vi "AlliGator Script Multi-ROI Single-Pixel Phasor Analysis.vi"(0 "Alligator Queue Elements in":T23[](array[typedef]), 1 "IRF File":path, 2 "Dataset File":path, 3 "ROI File":path, 5 "Error In":errorcluster, 6 "Phasor Graph refnum":refnum<vi>, 7 "Results Folder":path, 8 "Lifetime Graph Refnum":refnum<vi>, 10 "IRF Loading & Pre-processing Options":T4={"Data Information"={"Gates to Skip"={"Start"=0, "End"=0}, "# Gates"=1, "Gate Step"=1, "Gate Duration"=3e-10, "Gate Separation"=4e-11, "Pile-up Correction"=FALSE, "Pixel Well Capacity"=1, "Define Gates to"=enum."Skip", "Gates to Keep"={"First"=0, "Last"=0}, "Laser Period"=0.0, "SYNC Period"=0.0, "Channel Name"=0, "Channel Arithmetic"=enum."None", "Background File Subtraction"=FALSE, "Background Scaling Factor"=1.0, "Background File"=path "", "Background Pile-up Correction"=FALSE, "Background Pixel Well Capacity"=1, "Dataset Scaling Factor"=1.0}, "Source Image Settings"={"Low Count Pixels Rejection Options"={"Background Low Threshold Factor"=0.0, "Fixed Low Background Threshold"=20000.0, "Reject Low Count Pixels"=FALSE, "Low Percentile"=0.0}, "High Count Pixels Rejection Options"={"Background High Threshold Factor"=0.0, "Fixed High Background Threshold"=1.0, "Reject High Count Pixels"=FALSE, "High Percentile"=100.0}, "Peak Threshold"=500.0, "Intensity Threshold"=500.0, "Image Smoothing Options"={"Use Image Smoothing"=FALSE, "Kernel Type"=enum."Bilinear", "Bin"=1, "Algorithm"=enum."Rapid"}, "Image Binning Options"={"Use Image Binning"=FALSE, "X Bin"=1, "Y Bin"=1}}, "Decay Preprocessing Options & Parameters"={"Background Subtraction Parameters"={"Background Definition Range"={"Min Gate"=0.0, "Max Gate"=0.0}, "Baseline Subtraction Method"=enum."Mean", "Background Subtraction?"=FALSE, "Background File"=path "", "Background Constant"=0.0, "Background Scaling Factor"=1.0, "Background Pile-up Correction"=FALSE, "Background Pixel Well Capacity"=1}, "Decay Preprocessing Parameters"={"Background Subtraction"=FALSE, "Straighten Decay"=FALSE, "Reverse Gates"=FALSE, "1-Normalized Decay"=FALSE, "Smoothen Decay"=FALSE, "Smoothing Parameter"=0.0, "Shift Decay"=FALSE, "Decay Shift Parameters"={"Type"=enum."Default", "Shift"=0.0, "Threshold"=0.0, "Rotate"=FALSE}, "Extrapolate Decay"=FALSE, "Additional Points"=0, "Head Fraction"=0.0, "Pixel-Normalize Decay"=FALSE, "Use Periodicity"=FALSE, "Use Cursors"=FALSE, "Tail Fraction"=0.0, "Use Decay Pre-Processing"=TRUE, "Fold Decay"=FALSE, "# Folds"=1, "[0-1]-Normalized Decay"=FALSE}, "Preprocessing Steps Order"=[]}, "Clear Phasor Graph"=FALSE} {"Decay Preprocessing Options & Parameters"."Decay Preprocessing Parameters"."# Folds" min=1; "Decay Preprocessing Options & Parameters"."Background Subtraction Parameters"."Background Pixel Well Capacity" min=1 step=1; "Source Image Settings"."Image Binning Options"."Y Bin" min=1; "Source Image Settings"."Image Binning Options"."X Bin" min=1; "Source Image Settings"."Image Smoothing Options"."Bin" min=1; "Source Image Settings"."High Count Pixels Rejection Options"."High Percentile" min=0.0 max=100.0; "Source Image Settings"."Low Count Pixels Rejection Options"."Low Percentile" min=0.0 max=100.0; "Data Information"."Background Pixel Well Capacity" min=1 step=1; "Data Information"."Channel Name" items=["Bottom INT Gate", "Bottom G2 Gate"]; "Data Information"."SYNC Period" min=0.0 format="%#.3g"; "Data Information"."Laser Period" min=0.0 format="%#.3g"; "Data Information"."Pixel Well Capacity" min=1 step=1; "Data Information"."# Gates" min=1 step=1; "Data Information"."Gate Step" min=1 step=1; "Data Information"."Gate Duration" min=0.0 format="%#.3g"; "Data Information"."Gate Separation" min=0.0 format="%#.3g"}, 11 "Phasor Parameters Scatter Plot":T1[](array[typedef]), 12 "Dataset Loading & Pre-processing Options":T4={"Data Information"={"Gates to Skip"={"Start"=0, "End"=0}, "# Gates"=1, "Gate Step"=1, "Gate Duration"=3e-10, "Gate Separation"=4e-11, "Pile-up Correction"=FALSE, "Pixel Well Capacity"=1, "Define Gates to"=enum."Skip", "Gates to Keep"={"First"=0, "Last"=0}, "Laser Period"=0.0, "SYNC Period"=0.0, "Channel Name"=0, "Channel Arithmetic"=enum."None", "Background File Subtraction"=FALSE, "Background Scaling Factor"=1.0, "Background File"=path "", "Background Pile-up Correction"=FALSE, "Background Pixel Well Capacity"=1, "Dataset Scaling Factor"=1.0}, "Source Image Settings"={"Low Count Pixels Rejection Options"={"Background Low Threshold Factor"=0.0, "Fixed Low Background Threshold"=20000.0, "Reject Low Count Pixels"=FALSE, "Low Percentile"=0.0}, "High Count Pixels Rejection Options"={"Background High Threshold Factor"=0.0, "Fixed High Background Threshold"=1.0, "Reject High Count Pixels"=FALSE, "High Percentile"=100.0}, "Peak Threshold"=500.0, "Intensity Threshold"=500.0, "Image Smoothing Options"={"Use Image Smoothing"=FALSE, "Kernel Type"=enum."Bilinear", "Bin"=1, "Algorithm"=enum."Rapid"}, "Image Binning Options"={"Use Image Binning"=FALSE, "X Bin"=1, "Y Bin"=1}}, "Decay Preprocessing Options & Parameters"={"Background Subtraction Parameters"={"Background Definition Range"={"Min Gate"=0.0, "Max Gate"=0.0}, "Baseline Subtraction Method"=enum."Mean", "Background Subtraction?"=FALSE, "Background File"=path "", "Background Constant"=0.0, "Background Scaling Factor"=1.0, "Background Pile-up Correction"=FALSE, "Background Pixel Well Capacity"=1}, "Decay Preprocessing Parameters"={"Background Subtraction"=FALSE, "Straighten Decay"=FALSE, "Reverse Gates"=FALSE, "1-Normalized Decay"=FALSE, "Smoothen Decay"=FALSE, "Smoothing Parameter"=0.0, "Shift Decay"=FALSE, "Decay Shift Parameters"={"Type"=enum."Default", "Shift"=0.0, "Threshold"=0.0, "Rotate"=FALSE}, "Extrapolate Decay"=FALSE, "Additional Points"=0, "Head Fraction"=0.0, "Pixel-Normalize Decay"=FALSE, "Use Periodicity"=FALSE, "Use Cursors"=FALSE, "Tail Fraction"=0.0, "Use Decay Pre-Processing"=TRUE, "Fold Decay"=FALSE, "# Folds"=1, "[0-1]-Normalized Decay"=FALSE}, "Preprocessing Steps Order"=[]}, "Clear Phasor Graph"=FALSE} {"Decay Preprocessing Options & Parameters"."Decay Preprocessing Parameters"."# Folds" min=1; "Decay Preprocessing Options & Parameters"."Background Subtraction Parameters"."Background Pixel Well Capacity" min=1 step=1; "Source Image Settings"."Image Binning Options"."Y Bin" min=1; "Source Image Settings"."Image Binning Options"."X Bin" min=1; "Source Image Settings"."Image Smoothing Options"."Bin" min=1; "Source Image Settings"."High Count Pixels Rejection Options"."High Percentile" min=0.0 max=100.0; "Source Image Settings"."Low Count Pixels Rejection Options"."Low Percentile" min=0.0 max=100.0; "Data Information"."Background Pixel Well Capacity" min=1 step=1; "Data Information"."Channel Name" items=["Bottom INT Gate", "Bottom G2 Gate"]; "Data Information"."SYNC Period" min=0.0 format="%#.3g"; "Data Information"."Laser Period" min=0.0 format="%#.3g"; "Data Information"."Pixel Well Capacity" min=1 step=1; "Data Information"."# Gates" min=1 step=1; "Data Information"."Gate Step" min=1 step=1; "Data Information"."Gate Duration" min=0.0 format="%#.3g"; "Data Information"."Gate Separation" min=0.0 format="%#.3g"}) -> (14 "Alligator Queue Elements out":T23[](array[typedef]), 17 "Message":string, 19 "Error Out":errorcluster)   [LabVIEW 2021, in "AlliGator Scripts.lvlib"]
doc: "Scripts performing phasor analysis of all pixels in all ROIs, using individual IRFs if provided."
uses:
  AlliGator Scripts.lvlib
  Action Engine/AlliGator Q Event.ctl
  Action Engine/AlliGator Action Engine.lvlib
  Action Engine/AlliGator Q Element.ctl
  Action Engine/Alligator Elements Order in Action Stack.ctl
  Strings/Strings.lvlib
  Action Engine/AlliGator Add Action Array to Stack.vi
  Globals, Variables, Constants/AlliGator Globals, Variables & Constants.lvlib
  Globals, Variables, Constants/AlliGator Variables List.ctl
  Phasor/Phasor Calibration Type.ctl
  Phasor/Phasor.lvlib
  Files/Load-Save File Info.ctl
  Files/Files.lvlib
  <vilib>/Utility/miscctls.llb/LVPoint32TypeDef.ctl
  Graphs/XY Graph/XY Graph Refnum.ctl
  Graphs/XY Graph/XY Graph Add-Ons.lvlib
  Graphs/XY Graph/XY Graph Mouse Click Event Data.ctl
  Settings/AlliGator Settings.lvlib
  Action Engine/AlliGator Add Single Action to Stack.vi
  Graphs/XY Graph/XY Graph Save Plot Data.ctl
  Graphs/XY Graph/XY Graph Selected Plot Info.ctl
  Phasor Graph/AlliGator Phasor Graph.lvlib
  <vilib>/ErrorRing/Error Ring.xnode
  <vilib>/Utility/error.llb/Error Cluster From Error Code.vi
  ROIs/AlliGator ROIs.lvlib
  Graphs/Graphs.lvlib
  Settings/AlliGator Background Subtraction Parameters.ctl
  Settings/AlliGator Gates to Keep.ctl
  AlliGator Data Information.ctl
  Settings/AlliGator Low Count Pixels Rejection Options.ctl
  Settings/AlliGator High Count Pixels Rejection Options.ctl
  Arrays/Kernel Type.ctl
  Arrays/Arrays.lvlib
  Arrays/Smoothing Algorithm.ctl
  Settings/AlliGator Image Smoothing Options.ctl
  Source Image/AlliGator Image Binning Options.ctl
  Source Image/AlliGator Source Image.lvlib
  AlliGator Source Image Settings.ctl
  Decay Analysis/Decay Preprocessing/AlliGator Baseline Subtraction Method.ctl
  Decay Analysis/Decay Preprocessing/AlliGator Decay Preprocessing.lvlib
  Decay Analysis/Decay Preprocessing/AlliGator Background Subtraction Parameters.ctl
  Graphs/XY Graph/XY Graph Plot Shift Method.ctl
  Graphs/XY Graph/XY Graph Plot Shift Parameters.ctl
  Decay Analysis/Decay Preprocessing/AlliGator Decay Preprocessing Parameters.ctl
  Decay Analysis/Decay Preprocessing/AlliGator Decay Preprocessing Options.ctl
  AlliGator Data Load & Process Options.ctl
  Settings/AlliGator Gate Arithmetic.ctl
  Phasor Graph/AlliGator Phasor Graph Parameter List.ctl
  Phasor Graph/AlliGator Phasor Plot Scatter Plot Parameters.ctl
  Settings/AlliGator Define Gates to.ctl
panel:
  in  "Tab Control":T3(tab)
  # "see the AlliGator License on the block diagram (Ctrl+E or Window:Show Block Diagram)"
  # "vs"
  # "Gates Characteristics"
  # "Background File Subtraction"
  # "Gates Characteristics"
  # "Background File Subtraction"
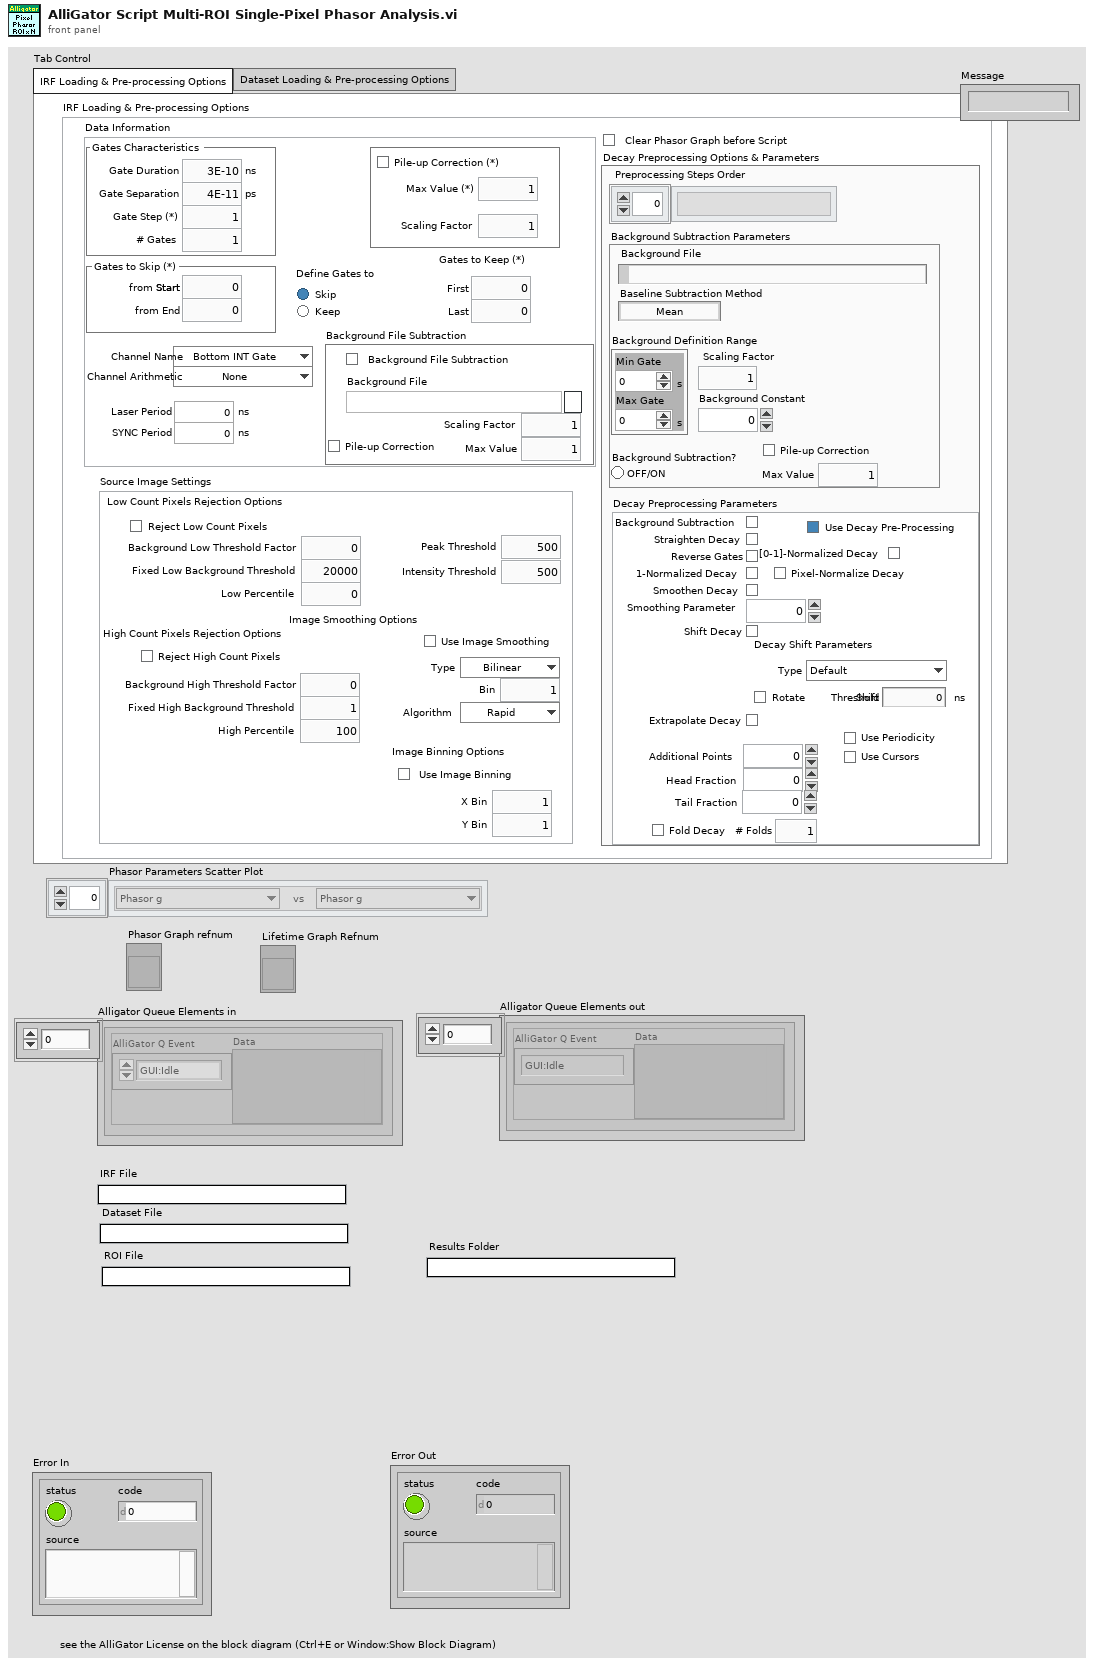
[diagram p1: front panel]
types:
  T1 = typedef "AlliGator Phasor Graph.lvlib/AlliGator Phasor Plot Scatter Plot Parameters.ctl" = cluster{"Parameter 2":T2, "Parameter 1":T2}
  T2 = typedef "AlliGator Phasor Graph.lvlib/AlliGator Phasor Graph Parameter List.ctl" = enum16{"Time Stamp", "Index", "Phasor Parameters", "Phasor g", "Phasor s", "Phasor phi", "Phasor m", "Modulus Lifetime", "Phase Lifetime", "ROI Parameters", "ROI Center x", "ROI Center y", "ROI # pixels ", "Decay Parameters", "Intensity", "Background/Gate", "Intensity - Background", "Fitted Lifetime", "Fitted Intensity", "Phasor Ratio Parameters", "Amplitude Phasor Ratio", "Intensity Phasor Ratio", "Amplitude-Averaged Lifetime", "Intensity-Averaged Lifetime", "-", "Phasor Parameters SDV", "Phasor g SDV", "Phasor s SDV", "Phasor phi SDV", "Phasor m SDV", "Phase Lifetime SDV", "Modulus Lifetime SDV", "Phasor Ratio Parameters SDV", "Amplitude Phasor Ratio SDV", "Intensity Phasor Ratio SDV", "Amplitude-Averaged Lifetime SDV", "Intensity-Averaged Lifetime SDV"}
  T3 = enum32{"IRF Loading & Pre-processing Options", "Dataset Loading & Pre-processing Options"}
  T4 = typedef "AlliGator Scripts.lvlib/AlliGator Data Load & Process Options.ctl" = cluster{"Data Information":T5, "Source Image Settings":T10, "Decay Preprocessing Options & Parameters":T17, "Clear Phasor Graph":bool}
  T5 = typedef "AlliGator Scripts.lvlib/AlliGator Data Information.ctl" = cluster{"Gates to Skip":T6, "# Gates":u32, "Gate Step":u32, "Gate Duration":dbl[unit], "Gate Separation":dbl[unit], "Pile-up Correction":bool, "Pixel Well Capacity":u32, "Define Gates to":T7, "Gates to Keep":T8, "Laser Period":dbl[unit], "SYNC Period":dbl[unit], "Channel Name":u16, "Channel Arithmetic":T9, "Background File Subtraction":bool, "Background Scaling Factor":dbl, "Background File":path, "Background Pile-up Correction":bool, "Background Pixel Well Capacity":u32, "Dataset Scaling Factor":dbl}
  T6 = typedef "AlliGator Settings.lvlib/AlliGator Background Subtraction Parameters.ctl" = cluster{"Start":u32, "End":u32}
  T7 = typedef "AlliGator Settings.lvlib/AlliGator Define Gates to.ctl" = enum32{"Skip", "Keep"}
  T8 = typedef "AlliGator Settings.lvlib/AlliGator Gates to Keep.ctl" = cluster{"First":u32, "Last":u32}
  T9 = typedef "AlliGator Settings.lvlib/AlliGator Gate Arithmetic.ctl" = enum16{"None", "INT-G2", "G2/INT*<INT>", "(1 - G2/INT)*<INT>"}
  T10 = typedef "AlliGator Scripts.lvlib/AlliGator Source Image Settings.ctl" = cluster{"Low Count Pixels Rejection Options":T11, "High Count Pixels Rejection Options":T12, "Peak Threshold":dbl, "Intensity Threshold":dbl, "Image Smoothing Options":T13, "Image Binning Options":T16}
  T11 = typedef "AlliGator Settings.lvlib/AlliGator Low Count Pixels Rejection Options.ctl" = cluster{"Background Low Threshold Factor":dbl, "Fixed Low Background Threshold":dbl, "Reject Low Count Pixels":bool, "Low Percentile":dbl}
  T12 = typedef "AlliGator Settings.lvlib/AlliGator High Count Pixels Rejection Options.ctl" = cluster{"Background High Threshold Factor":dbl, "Fixed High Background Threshold":dbl, "Reject High Count Pixels":bool, "High Percentile":dbl}
  T13 = typedef "AlliGator Settings.lvlib/AlliGator Image Smoothing Options.ctl" = cluster{"Use Image Smoothing":bool, "Kernel Type":T14, "Bin":i32, "Algorithm":T15}
  T14 = typedef "Arrays.lvlib/Kernel Type.ctl" = enum16{"Uniform", "Bilinear", "Gaussian"}
  T15 = typedef "Arrays.lvlib/Smoothing Algorithm.ctl" = enum16{"Rapid", "Thorough"}
  T16 = typedef "AlliGator Source Image.lvlib/AlliGator Image Binning Options.ctl" = cluster{"Use Image Binning":bool, "X Bin":i32, "Y Bin":i32}
  T17 = typedef "AlliGator Decay Preprocessing.lvlib/AlliGator Decay Preprocessing Options.ctl" = cluster{"Background Subtraction Parameters":T18, "Decay Preprocessing Parameters":T20, "Preprocessing Steps Order":string[]}
  T18 = typedef "AlliGator Decay Preprocessing.lvlib/AlliGator Background Subtraction Parameters.ctl" = cluster{"Background Definition Range":cluster{"Min Gate":dbl[unit], "Max Gate":dbl[unit]}, "Baseline Subtraction Method":T19, "Background Subtraction?":bool, "Background File":path, "Background Constant":dbl, "Background Scaling Factor":dbl, "Background Pile-up Correction":bool, "Background Pixel Well Capacity":u32}
  T19 = typedef "AlliGator Decay Preprocessing.lvlib/AlliGator Baseline Subtraction Method.ctl" = enum16{"Mean", "Min", "Square Gated Single-Exponential", "File", "Constant"}
  T20 = typedef "AlliGator Decay Preprocessing.lvlib/AlliGator Decay Preprocessing Parameters.ctl" = cluster{"Background Subtraction":bool, "Straighten Decay":bool, "Reverse Gates":bool, "1-Normalized Decay":bool, "Smoothen Decay":bool, "Smoothing Parameter":dbl, "Shift Decay":bool, "Decay Shift Parameters":T21, "Extrapolate Decay":bool, "Additional Points":u32, "Head Fraction":dbl, "Pixel-Normalize Decay":bool, "Use Periodicity":bool, "Use Cursors":bool, "Tail Fraction":dbl, "Use Decay Pre-Processing":bool, "Fold Decay":bool, "# Folds":u32, "[0-1]-Normalized Decay":bool}
  T21 = typedef "XY Graph Add-Ons.lvlib/XY Graph Plot Shift Parameters.ctl" = cluster{"Type":T22, "Shift":dbl[unit], "Threshold":dbl, "Rotate":bool}
  T22 = typedef "XY Graph Add-Ons.lvlib/XY Graph Plot Shift Method.ctl" = enum16{"Default", "CFD", "Threshold", "Cross-Correlation"}
  T23 = typedef "AlliGator Action Engine.lvlib/AlliGator Q Element.ctl" = cluster{"AlliGator Q Event":T24, "Data":variant}
  T24 = typedef "AlliGator Action Engine.lvlib/AlliGator Q Event.ctl" = enum16{"---- Files ----", "Files:Set Batch Export Files To Save", "Files:Set Dataset Loading & Pre-processing Options", "Files:Check #Frames in Dataset", "Files:Increment Frame Index", "Files:Open Mask Image", "Files:Open White Light Image", "Files:Open Single Dataset", "Files:New Folder of Folders Selected", "Files:Load File (all Types)_Scriptable", "Files:Move Flattened Series to Folders Series", "Files:Select Folder", "Files:Load FLI Dataset", "Files:Load Swiss SPAD 1 Dataset", "Files:Load Swiss SPAD 2 Dataset", "Files:Load .sdt FLI Dataset", "Files:Load .ptu FLI Dataset", "Files:Load .bin FLI Dataset", "Files:Load Single Gate Image Folder", "Files:Load I/m/phi Dataset (deprecated)", "Files:Load Single Image", "Files:Subtract Background File", "Files:Export FLI Dataset", "Files:Load HDF5 FLI Dataset", "Files:Set Destination File Path", "Files:Save Mask Image", "Files:Batch Conversion", "Files:New Folder Selected", "Files:Close FLI Dataset", "Files:Close FLI Dataset Series", "Files:Close White Light Image", "Files:Close Mask Image", "---- FLI Dataset ----", "FLI Dataset:Channel Arithmetic", "FLI Dataset:Export Average Lifetime Map as ASCII", "FLI Dataset:Export User-Defined Quantity Map as ASCII", "FLI Dataset:Python Function FLI Dataset Event", "FLI Dataset:ROI Analysis", "FLI Dataset:Tilted Logistic Square Gated IRF Characteristics Map", "FLI Dataset:Logistic Square Gated IRF Characteristics Map", "FLI Dataset:Square Gated IRF Characteristics Map", "FLI Dataset:Multi-ROI Single-Pixel Phasor Analysis", "FLI Dataset:Multi-ROI Single-Pixel NLSF Analysis", "FLI Dataset:All ROIs IRF Extraction", "FLI Dataset:All ROIs Decay Fit Non-Interactive (Fast + Individual IRF)", "FLI Dataset:All ROIs Phasor Analysis", "FLI Dataset:All ROIs Decay Fit", "FLI Dataset:Fluorescence Decay Statistics", "FLI Dataset:Update Decay Statistics Graph", "FLI Dataset:Get Decay from ROI", "FLI Dataset:All ROIs Average Lifetimes", "---- FLI Dataset Series ----", "FLI Dataset Series:Sum All Datasets in Series", "FLI Dataset Series:Add Dataset to Accumulated Dataset", "FLI Dataset Series:Display Accumulated Dataset", "FLI Dataset Series:Clear Dataset Series Sum", "FLI Dataset Series:Time-Series Analysis (NLSF)", "FLI Dataset Series:Time-Series Analysis (Phasor)", "---- Image ----", "Image:Update Image Profile Plots", "Image:Image Histogram Cursor Move", "Image:Image Histogram", "Image:Image Contrast", "Image:Set Image Histogram Cursor Move Flag", "Image:Clear Image Overlay", "Image:Use ROI as Search Area", "Image:Set ROI Diameter", "Image:Save Image Data as TIFF", "Image:Save Displayed Image with Overlay", "Image:Save Image Overlay Only", "Image:Save Image as Hot Pixel Mask", "Image:Change Source Image Color Palette", "Image:Copy Image to Clipboard", "Image:Source Image ROI Selection", "Image:Delete All ROIs", "Image:Delete All Unselected ROIs", "Image:Delete ROI", "Image:Merge All ROIs", "Image:Store ROI", "Image:Source Image ROI Storage", "Image:Export ROI Description to Notebook", "Image:Save ROI", "Image:Load ROI", "Image:Paste ROI Definition", "Image:Clear ROI", "Image:Identify ROIs in Mask Image", "Image:Create Complementary ROI", "Image:Create Contour ROI", "Image:Create ROI(s) from Pixels with Peak above Min_Scriptable", "Image:Create ROI(s) from Pixels with Intensity above Min_Scriptable", "Image:Compute ROI Statistics", "Image:Delete ROI(s) based on ROI Characteristics", "Image:Create ROI Grid", "Image:ROI to Individual Pixel ROIs", "Image:Python Function Source Image Event", "Image:Show Phasor Calibration Map ROI Centers", "Image:Convert ROI to Mask Image", "Image:Mouse Move", "Image:Mouse Up", "Image:Set Source Image Mouse Move Flag", "Image:Add Scale Bar Overlay", "Image:Delete Existing ROIs Option", "Image:Overlay ROI Median", "Image:Check Current ROI", "---- Decay ----", "Decay:Clear IRF/Reference Plot", "Decay:Clear Local IRFs", "Decay:Add Decay to Graph", "Decay:Smoothen Plot", "Decay:Smoothen Plot Tail", "Decay:Average Selected Plots", "Decay:Extract IRF", "Decay:Optimal IRF Extraction", "Decay:Threshold IRF", "Decay:Fit to Model IRF", "Decay:Fit IRF to Square Gate", "Decay:Fit IRF to Logistic Square Gate", "Decay:Fit IRF to Tilted Logistic Square Gate", "Decay:Create Bounding Cursors Set", "Decay:Export Bounding Cursors Definition to Notebook", "Decay:Denoise Plot", "Decay:Compute Cumulative Function", "Decay:Use as Reference Decay", "Decay:Show Reference Decay/IRF", "Decay:Extrapolate Decay", "Decay:Create Head & Tail Bounding Cursors", "Decay:Store Cursor-defined Head & Tail Fractions", "Decay:Rebin Plot", "Decay:1-Normalize Decay", "Decay:[0-1]-Normalize Plot", "Decay:Straighten Decay", "Decay:Shift Decay", "Decay:Fold Decay", "Decay:Fit Decay", "Decay:Global Fit of Selected Decays", "Decay:Post Global Fit Script", "Decay:Add Global Fit Parameters to Graph", "Decay:Add Decay Parameter(s) to Plot (Graph)", "Decay:Export Decay to Phasor Graph", "Decay:Plot Decay Shifts", "Decay:Compute Average Lifetime", "Decay:Plot Convolution", "Decay:Graph Tip Strip Update", "---- Decay Statistics ----", "Decay Statistics:Tip Strip Update", "---- Intensity Time Trace ----", "Intensity Time Trace:Use File Timestamp", "Intensity Time Trace:Load Intensity Corrections File", "Intensity Time Trace:Clear Intensity Corrections File", "Intensity Time Trace:Tip Strip Update", "---- Phasor Plot ----", "Phasor Plot:Build Phasor Plot", "Phasor Plot:Change Phasor Plot Color Palette", "Phasor Plot:Adjust Phasor Plot Display Range", "Phasor Plot:Highlight Image ROI in Phasor Plot", "Phasor Plot:Save Phasor Plot Image with Overlay", "Phasor Plot:Export Complex Phasor Map", "Phasor Plot:Export Phasor Ratio Map", "Phasor Plot:Export Average Lifetime Map", "Phasor Plot:Compute Phase Lifetime Histogram", "Phasor Plot:Compute Phasor Ratio Histogram", "Phasor Plot:Compute Phase Lifetime vs Intensity Scatter Plot", "Phasor Plot:Weber 2-Component Decomposition", "Phasor Plot:Update Phasor Color Map Vertices", "Phasor Plot:Clear Phasor Overlay", "Phasor Plot:Use Segment Extremities as References", "Phasor Plot:Use UC/Segment Intersections as References", "Phasor Plot:Use UC/Principal Axis Intersections as References", "Phasor Plot:Use UC/Linear Fit Intersections as References", "Phasor Plot:Update Phasor Plot Reference", "Phasor Plot:Show Local Phasor Info in Phasor Plot", "Phasor Plot:Update Phasor Plot State", "Phasor Plot:Phasor Plot ROI Storage", "Phasor Plot:Phasor Plot ROI Selection", "Phasor Plot:Python Function Phasor Plot Event", "Phasor Plot:Overlay Phasor ROI, Ratio or Map in Source Image", "Phasor Plot:Compute Decay of Selected Phasors", "Phasor Plot:Phasor at Image Pixel", "Phasor Plot:Mouse Move", "Phasor Plot:Mouse Up", "Phasor Plot:Display Range Mouse Move", "Phasor Plot:Set Mouse Move Flag", "---- Phasor Graph ----", "Phasor Graph:Calibrated Phasor Map Series", "Phasor Graph:Whole Image Phasor Scatter Plot (deprecated)", "Phasor Graph:Get Phasor Value", "Phasor Graph:Create New Phasor Plot Dialog", "Phasor Graph:Update Last Phasor Value", "Phasor Graph:Update Phasor (m, phi)", "Phasor Graph:Remove Single Phasor from Plot", "Phasor Graph:Add Single Phasor to Plot", "Phasor Graph:Remove Phasor Plot", "Phasor Graph:Remove Selected Phasor Plots", "Phasor Graph:Clear Phasor Data", "Phasor Graph:Clear Phasor Graph", "Phasor Graph:Cursor Move", "Phasor Graph:Draw Cursor Connecting Line", "Phasor Graph:Clear Cursor Connecting Line", "Phasor Graph:Find UC Intersection", "Phasor Graph:Use UC/Cursor-Defined Line Intersections", "Phasor Graph:Use Selected Plots Fitted Line/UC Intersections", "Phasor Graph:Use Selected Plots Principal Axis/UC Intersections", "Phasor Graph:Show Single Phasor", "Phasor Graph:Save Single Phasor Plot", "Phasor Graph:Save All Phasor Plots", "Phasor Graph:Load Phasor Plot(s)", "Phasor Graph:Phasor Multiplication", "Phasor Graph:Compute Average Phasor", "Phasor Graph:Compute Multiple Average Phasors (Selected Plots)", "Phasor Graph:Export Single Phasor Plot Phase Lifetimes", "Phasor Graph:Phase Lifetime Trajectory (deprecated)", "Phasor Graph:Phase Lifetime vs Intensity Scatter Plot (deprecated)", "Phasor Graph:Parameter 2 vs Parameter 1 Scatter Plot", "Phasor Graph:Use Cursor n Location", "Phasor Graph:Set Reference n to Current Phase Lifetime Value", "Phasor Graph:Set Reference n to Lifetime Value", "Phasor Graph:Set Cursor n Location", "Phasor Graph:Save Phasor Graph Image", "Phasor Graph:Update SEPL Plot", "Phasor Graph:Export Single Phasor Plot Data", "Phasor Graph:Export Selected Phasor Plots Data", "Phasor Graph:Python Function Phasor Graph Event", "Phasor Graph:Tip Strip Update", "---- Calibration ----", "Calibration:Set Calibration Type", "Calibration:Load/Save Phasor Calibration", "Calibration:Load/Save Phasor Calibration Series", "Calibration:Load/Save Phasor Calibration Map", "Calibration:Use as Calibration", "Calibration:Compute Optimal Calibration from Phasor References", "Calibration:Clear Phasor Calibration", "Calibration:Single Phasor Calibration Information", "Calibration:Use as Calibration Series", "Calibration:Use as Calibration Map", "Calibration:Clear Calibration Series", "Calibration:Phasor Calibration Series Information", "Calibration:Clear Calibration Map", "Calibration:Phasor Calibration Map Information", "Calibration:Apply Phasor Calibration", "Calibration:Update Single Plot Calibration", "Calibration:Update Multiple Plots Calibration", "Calibration:Clear Single Plot Calibration", "Calibration:Clear All Plots Calibrations", "Calibration:Clear Plot(s) Calibration(s)?", "Calibration:Phasor Calibration Maps (# Gates Series)", "---- Phasor Ratio ----", "Phasor Ratio:Clear Reference n", "Phasor Ratio:Toggle Selected Plot(s)  Lock to Reference 1", "Phasor Ratio:Use as Reference n", "Phasor Ratio:Send Reference n to Notebook", "Phasor Ratio:Toggle Selected Plot(s)  Lock to Reference 2", "Phasor Ratio:Compute Phasor Ratio at Mouse Location", "Phasor Ratio:Compute Phasor Plot's Average Phasor Ratio", "Phasor Ratio:Compute Time-Series Phasor Ratios", "Phasor Ratio:Fit Line to Phasor Ratio Plot", "Phasor Ratio:Save References", "Phasor Ratio:Load References", "Phasor Ratio:Update Phasor Reference 1", "Phasor Ratio:Update Phasor Reference 2", "Phasor Ratio:Move Cursor n to Reference n", "Phasor Ratio:Use as Phasor Reference 1 Lifetime", "Phasor Ratio:Use as Phasor Reference 2 Lifetime", "Phasor Ratio:Export Phasor Ratio Map as ASCII", "Phasor Ratio:Tip Strip Update", "---- Lifetime & Other Parameters Graph ----", "Lifetime:Tip Strip Update", "---- Decay Fit Parameter Map ----", "Decay Fit Parameter Map:Export ROI NLSF Data as ASCII", "Decay Fit Parameter Map:Set Decay Fit Parameter Map Selection", "Decay Fit Parameter Map:Build Decay Fit Parameter Map", "Decay Fit Parameter Map:Change Decay Fit Parameter Map Color Palette", "Decay Fit Parameter Map:Export Decay Fit Parameter Map Data as ASCII", "Decay Fit Parameter Map:Export All Decay Fit Parameter Maps Data as ASCII", "Decay Fit Parameter Map:Selected Parameter Scatterplot", "Decay Fit Parameter Map:Parameter 2 vs Parameter 1 Scatterplot", "Decay Fit Parameter Map:Save Decay Fit Parameter Map Image", "Decay Fit Parameter Map:Save-Load IRFs & Fit Data", "Decay Fit Parameter Map:Update Local Decay Plots", "Decay Fit Parameter Map:Python Function Decay Fit Parameters Map Event", "Decay Fit Parameter Map:Overlay Decay Fit Parameter Map in Source Image", "Decay Fit Parameter Map:Selected Parameter vs Intensity Scatterplot", "Decay Fit Parameter Map:Mouse Up", "Decay Fit Parameter Map:Display Range Mouse Move", "---- Parameter Map ----", "Parameter Map:Export ROI Parameters Data as ASCII", "Parameter Map:Delete Parameter Map Set", "Parameter Map:Update Parameter List", "Parameter Map:Build Parameter Map", "Parameter Map:Change Parameter Map Color Palette", "Parameter Map:Export Parameter Map Data as ASCII", "Parameter Map:Export All Parameter Maps Data as ASCII", "Parameter Map:Selected Parameter Scatterplot", "Parameter Map:Parameter 2 vs Parameter 1 Scatterplot", "Parameter Map:Selected Parameter vs Intensity Scatterplot", "Parameter Map:Save Parameter Map Image", "Parameter Map:Save-Load IRFs & Parameter Maps (TODO)", "Parameter Map:Set Parameter Map Selection", "Parameter Map:Python Function Parameter Map Event", "Parameter Map:Overlay Parameter Map in Source Image", "Parameter Map:Update Local Decay Plots", "Parameter Map:Mouse Up", "Parameter Map:Display Range Mouse Move", "---- Generic Graph ----", "Generic Graph:Generic XY Graph Event", "Generic Graph:Python Function XY Graph Event", "Generic Graph:New Plot", "Generic Graph:Save Plot", "Generic Graph:XY Plot Histogram", "Generic Graph:Set XY Graph Plot Name", "Generic Graph:Set Last Cursor Style", "Generic Graph:Tip Strip Update", "---- GUI ----", "GUI:Start Script", "GUI:Type of Displayed Image Changed", "GUI:Gate Image Slide Changed", "GUI:Show Busy Icon", "GUI:Show Busy Icon & Abort Button", "GUI:Hide Busy Icon", "GUI:Hide Busy Icon & Abort Button", "GUI:Abort", "GUI:End Script", "GUI:Start Timing", "GUI:End Timing", "GUI:Set State Indicator", "GUI:Send Parameters JSON Strings to Clipboard", "GUI:Set Gate Step", "GUI:Idle", "GUI:Initialization", "GUI:Quit", "GUI:Increment Dataset Index", "GUI:Set Dataset Index to -1", "GUI:Time Series Slider Moved", "GUI:Time Series Slider Changed", "GUI:Toggle Playback or Loop", "GUI:Playback Script", "GUI:Set Phasor Frequency", "GUI:Open Window", "GUI:Start Test Script", "GUI:End Test Script", "DEBUG"}
  T25 = typedef "AlliGator Globals, Variables & Constants.lvlib/AlliGator Variables List.ctl" = enum16{"---- GUI ----", "GUI:Initialization Status", "GUI:State Indicators Refnum", "GUI:Original AlliGator Menu Items", "GUI:Current Action Loop State", "GUI:Script in progress", "GUI:Playback", "GUI:Loop Playback", "GUI:Search ROI Used", "GUI:Search ROI", "Decay Graph Max Legend Size", "Intensity Graph Max Legend Size", "Decay Statistics Graph Max Legend Size", "Phasor Graph Max Legend Size", "Phasor Ratio Graph Max Legend Size", "Lifetime Graph Max Legend Size", "---- Files ----", "Files:Export Dataset Frames as Individual Files", "Files:Show Batch Export Help Balloons", "Files:Frames in Dataset", "Files:ptu File Frame Start Indices", "Files:Current Frame in Dataset", "Files:Current Frame Timestamp", "Files:Dataset Loaded", "Files:Dataset Metadata", "Files:Dataset Channel", "Files:Dataset Data Description", "Files:Background Dataset Metadata", "Files:Background Dataset Channel", "Files:Background Dataset Data Description", "Files:Background File Subtraction", "Files:Background File Path", "Files:Background File Pile-up Correction", "Files:Background File Pixel Well Capacity", "Files:Background File Scaling Factor", "Files:Current Dataset Load Settings", "Files:Dataset Path", "Files:ICCD-specific Information", "Files:Macrotime Gate Separation", "------ Python Plugins ------", "Python Plugins:Information", "Python Plugins:Python Session", "Python Plugins:Valid Python Session?", "---- Source Image ----", "Source Image:ROIs", "Source Image:Current ROI", "Source Image:ROI Event Refnum", "X_Source Image Display Range", "X_Source Image Palette Information", "X_Type of Displayed Image", "X_Time Gate Slider", "Source Image:Palette List", "Source Image:Scale", "Source Image:ROI Overlay Color", "Source Image:Overlay to Erase", "Source Image:Is Displayed Image Accumulated", "Source Image:White Light Image Modified", "Source Image:Mask Image Modified", "---- Image Profile Window ----", "Image Profile:Window Event Refnum", "Image Profile:IntensityType", "Image Profile:Intensity Average Type", "Image Profile:Intensity-weighted SDV", "Image Profile:Box Profile Type", "Image Profile:Window Open", "Image Profile:Plotted Fit Parameter", "------ Phasor Graph -------", "Phasor Graph:Show Line", "---- Phasor Plot ---", "Phasor Plot:Parameters Changed", "Phasor Plot:FLI Dataset Modified since last Calculation", "Phasor Harmonics Data", "Selected Phasor Harmonics", "Phasor Harmonic Manager Event Refnum", "Phasor Plot:ROIs", "Phasor Plot:Current ROI", "Phasor Plot:ROI Event Refnum", "Phasor Plot:Image Reference Points", "Phasor Plot:Computed", "Phasor Plot:Palette Information", "Phasor Plot:Palette List", "Phasor Plot:Phasor Ratio Palette Information", "Phasor Plot:Phasor Ratio Palette List", "Phasor Plot:Image Scale", "Phasor Plot:Image Overlay to Erase", "Phasor Plot:Image Elements to Update", "Phasor Plot:Current Calculation Parameters", "Phasor Plot:Current Calibration Options", "Phasor Plot:Reset Cumulated Phasor Plot", "Phasor Plot:Reference 1", "Phasor Plot:Lifetime Reference 1", "Phasor Plot:Reference 1 Frequency", "Phasor Plot:Reference 2", "Phasor Plot:Lifetime Reference 2", "Phasor Plot:Reference 2 Frequency", "---- Decay Analysis ----", "Number of Selected Decays to Fit", "LS Fit Results", "LAR Fit Results", "BS Fit Results", "Last Decay Max - Min", "Best Fit Parameters", "Best Fit Parameter Names", "Actual Size X", "Actual Size Y", "Binning X", "Binning Y", "Actual # Gates", "Dataset Number", "Gates to...", "Gates Skipped", "Gates to keep", "Gate Step", "Gate Separation", "Reversed Gates", "Pile-up Correction", "Pixel Well Capacity", "Background Subtracted", "Background Subtraction Method", "Background Definition Range", "Background File (deprecated)", "Number of Dataset Accumulated", "Array of Accumulated Dataset Paths", "Do Averaged Datasets", "Destination File Path", "Process Plot Target", "Use 1/D as Phasor Frequency", "---- Decay Fit Parameter Map -----", "Decay Fit Parameter Map:Palette Information", "Decay Fit Parameter Map:Palette List", "---- Parameter Map ----", "Parameter Map:Palette Information", "Parameter Map:Palette List", "------- Local Decay Window ---------", "Local Decay Graph Window:Event Refnum", "Local Decay Graph Window:Use normalized IRF for convolution", "----- Miscellaneous ----", "Misc:Skippable Dialog Windows Status"}
  T26 = enum16{"Start Script", "Load & Analyze IRF Dataset", "Load & Analyse FLI Dataset: Phasor", "End Script"}
  T27 = typedef "AlliGator Action Engine.lvlib/Alligator Elements Order in Action Stack.ctl" = enum16{"Enqueue 2 AFTER 1", "Enqueue 2 BEFORE 1"}
  T28 = typedef "Phasor.lvlib/Phasor Calibration Type.ctl" = enum16{"None", "Single Phasor", "Phasor Series", "Phasor Map"}
  T29 = typedef "XY Graph Add-Ons.lvlib/XY Graph Mouse Click Event Data.ctl" = cluster{"Multiplot XY Graph":T30, "Mouse Coordinates":T31}
  T30 = typedef "XY Graph Add-Ons.lvlib/XY Graph Refnum.ctl" = refnum<vi>
  T31 = typedef "LVPoint32TypeDef.ctl" = cluster{"Horizontal":i32, "Vertical":i32}
  T32 = typedef "XY Graph Add-Ons.lvlib/XY Graph Selected Plot Info.ctl" = cluster{"Multiplot XY Graph":T30, "Mouse Coordinates":T31, "Plot Index":i32}
  T33 = typedef "XY Graph Add-Ons.lvlib/XY Graph Save Plot Data.ctl" = cluster{"XY Graph Refnum":refnum<vi>, "Mouse Coords":T31, "File Path":path}
  T34 = typedef "Files.lvlib/Load-Save File Info.ctl" = cluster{"Load/Save":bool, "File Path":path}
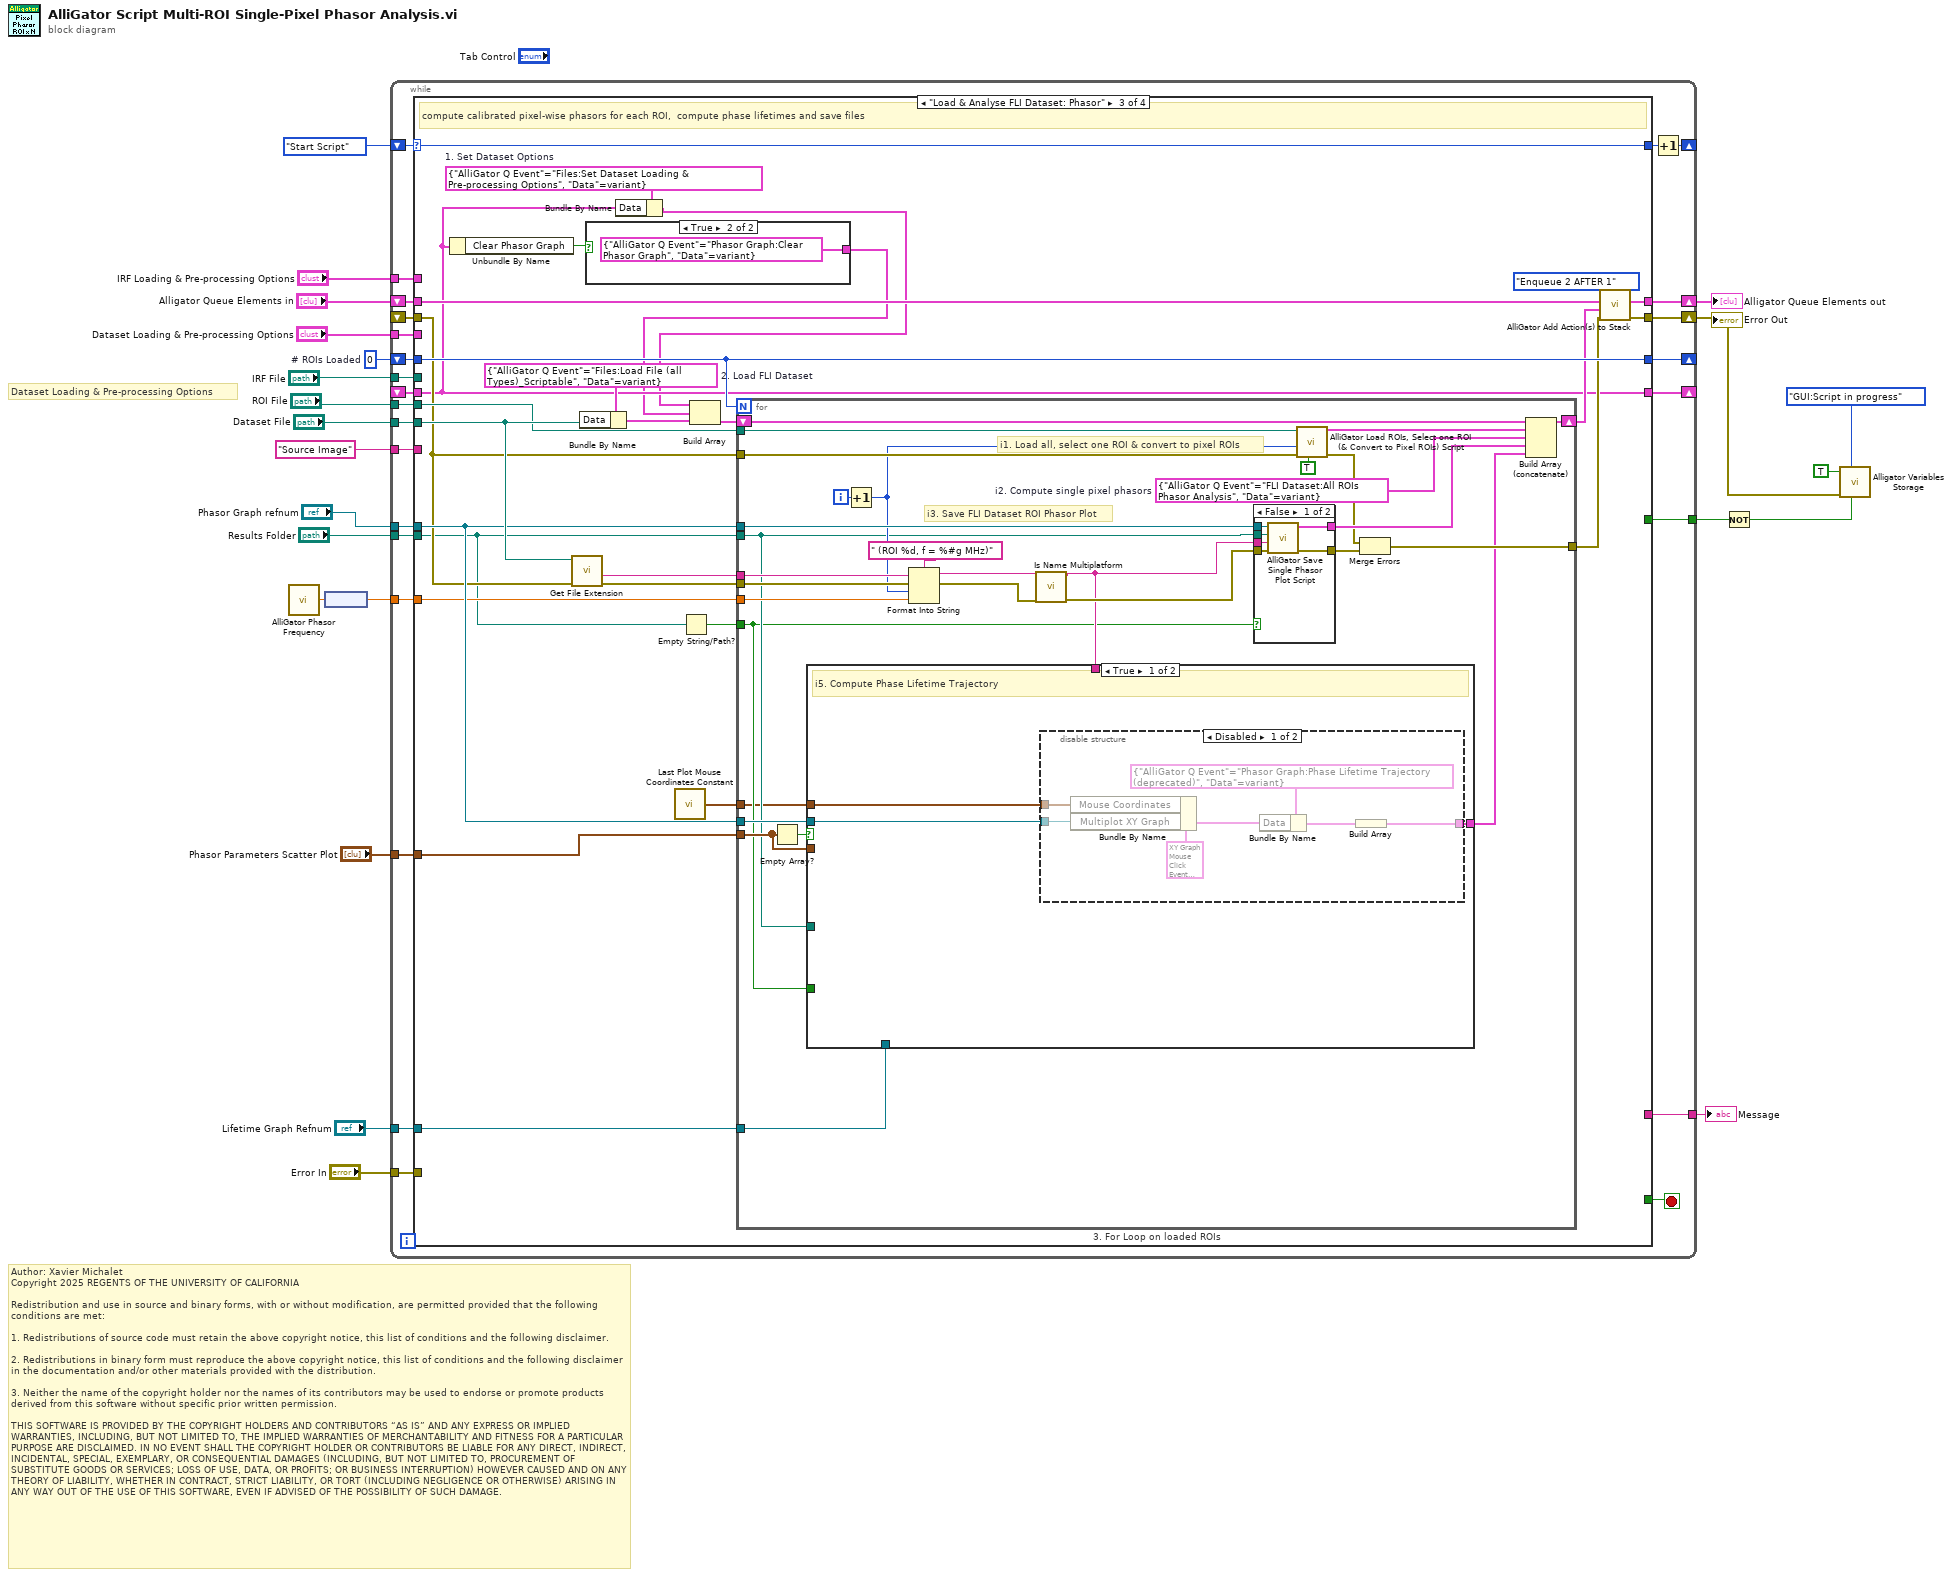
[diagram p0: block diagram]
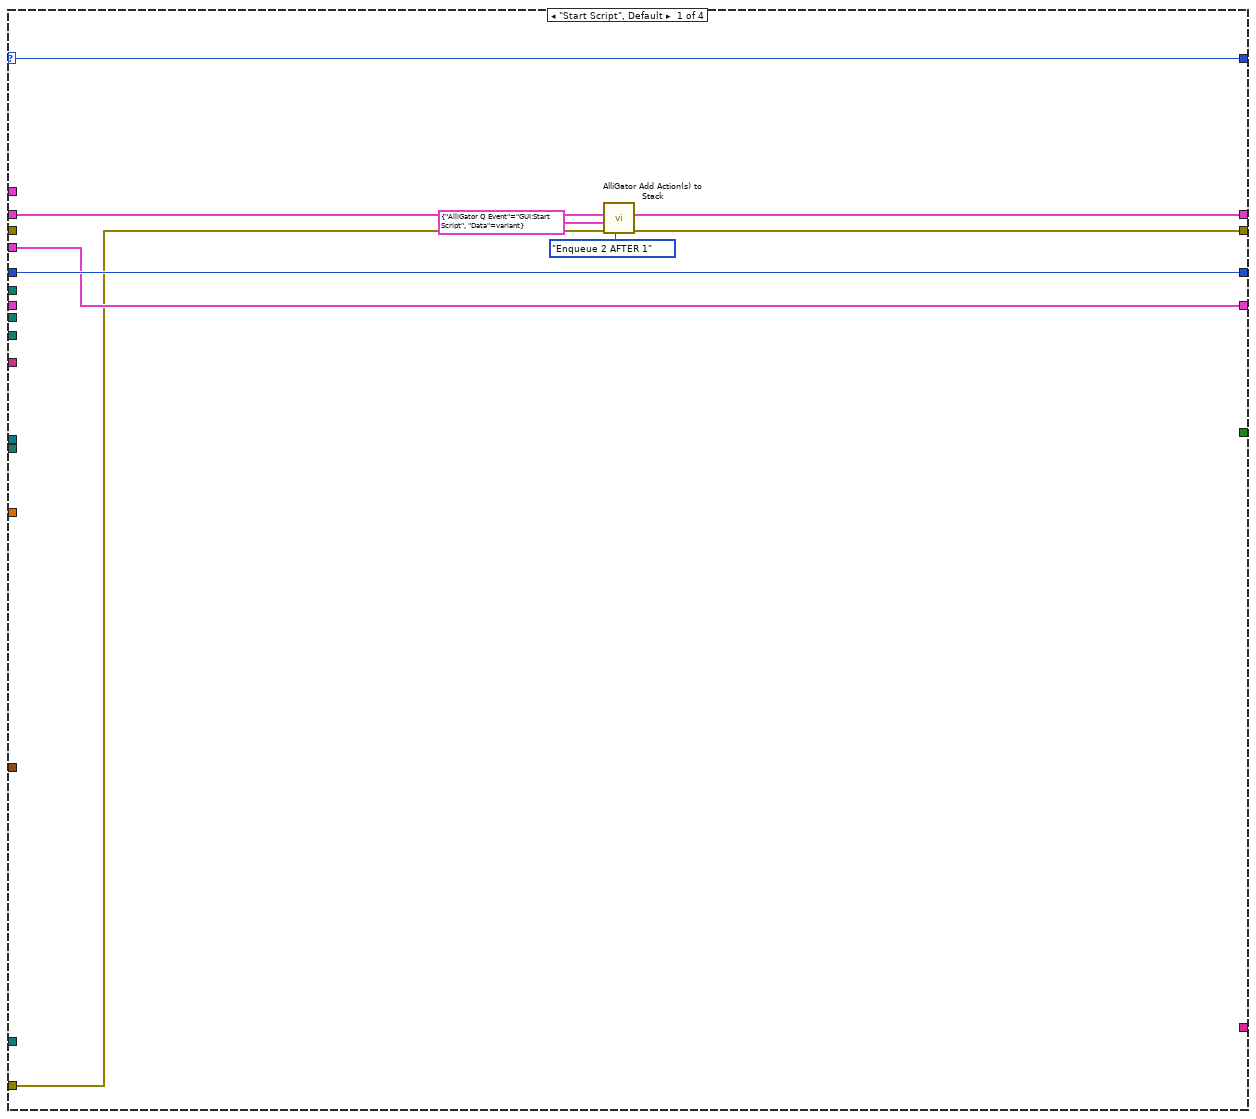
[diagram p2: hidden frame]
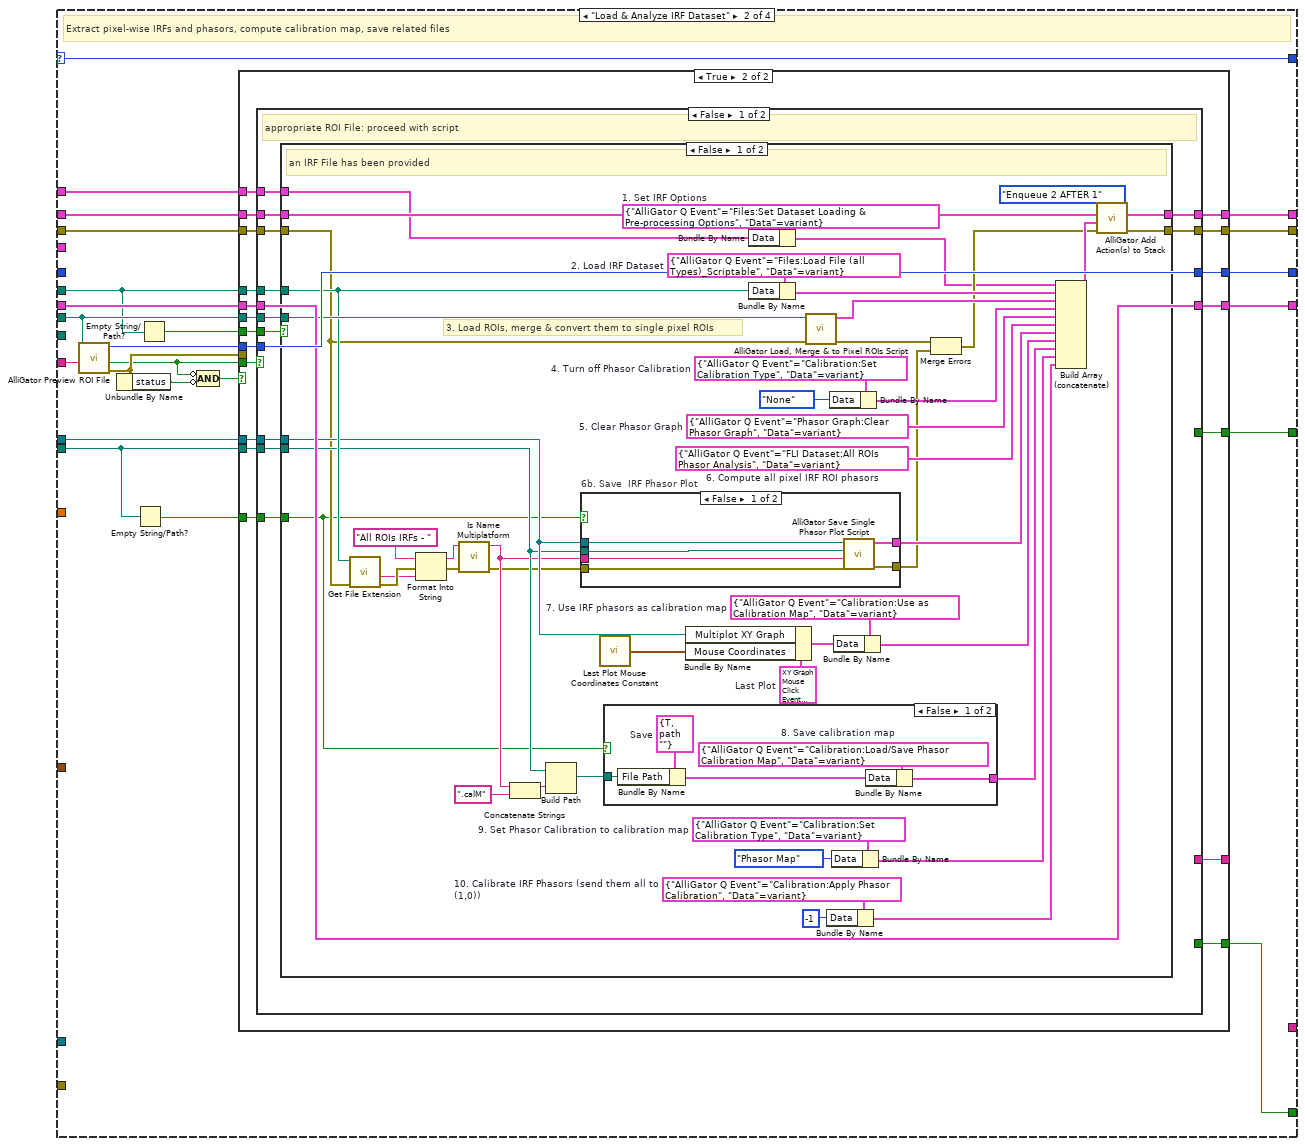
[diagram p3: hidden frame]
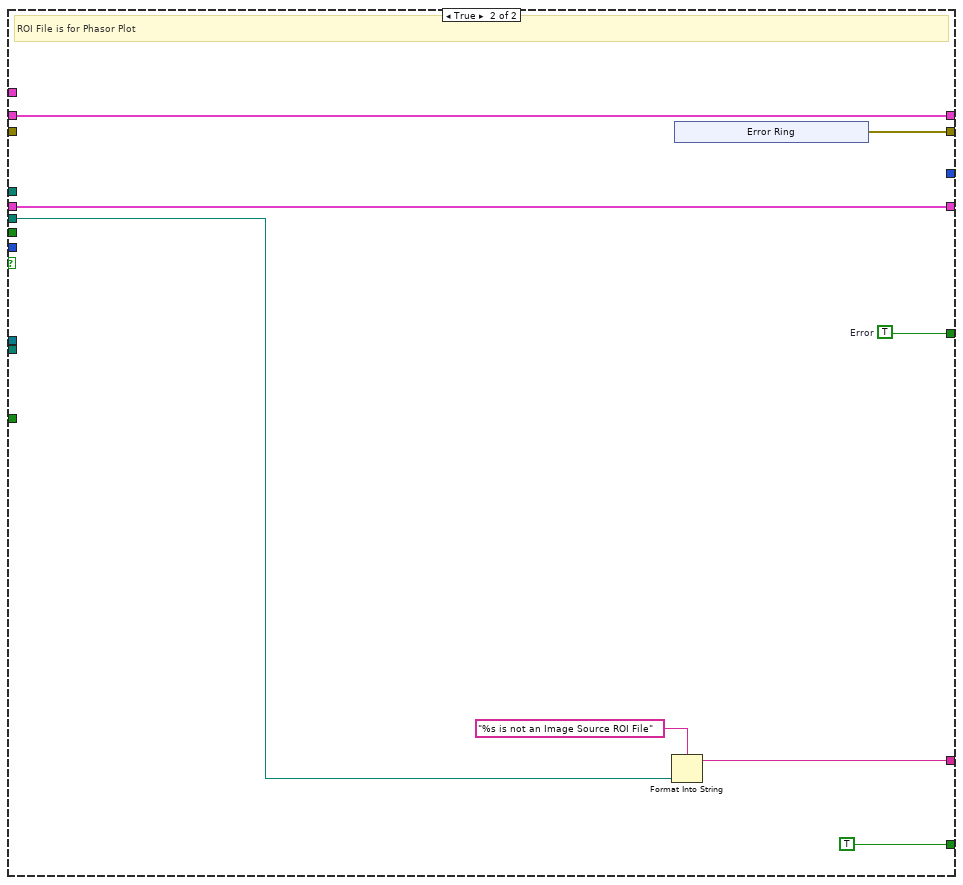
[diagram p8: hidden frame]
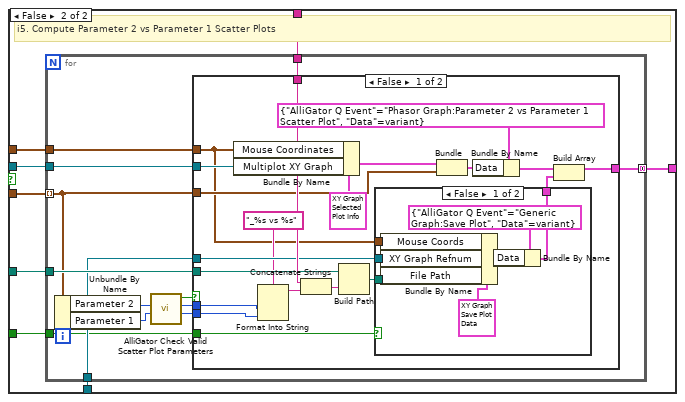
[diagram p11: hidden frame]
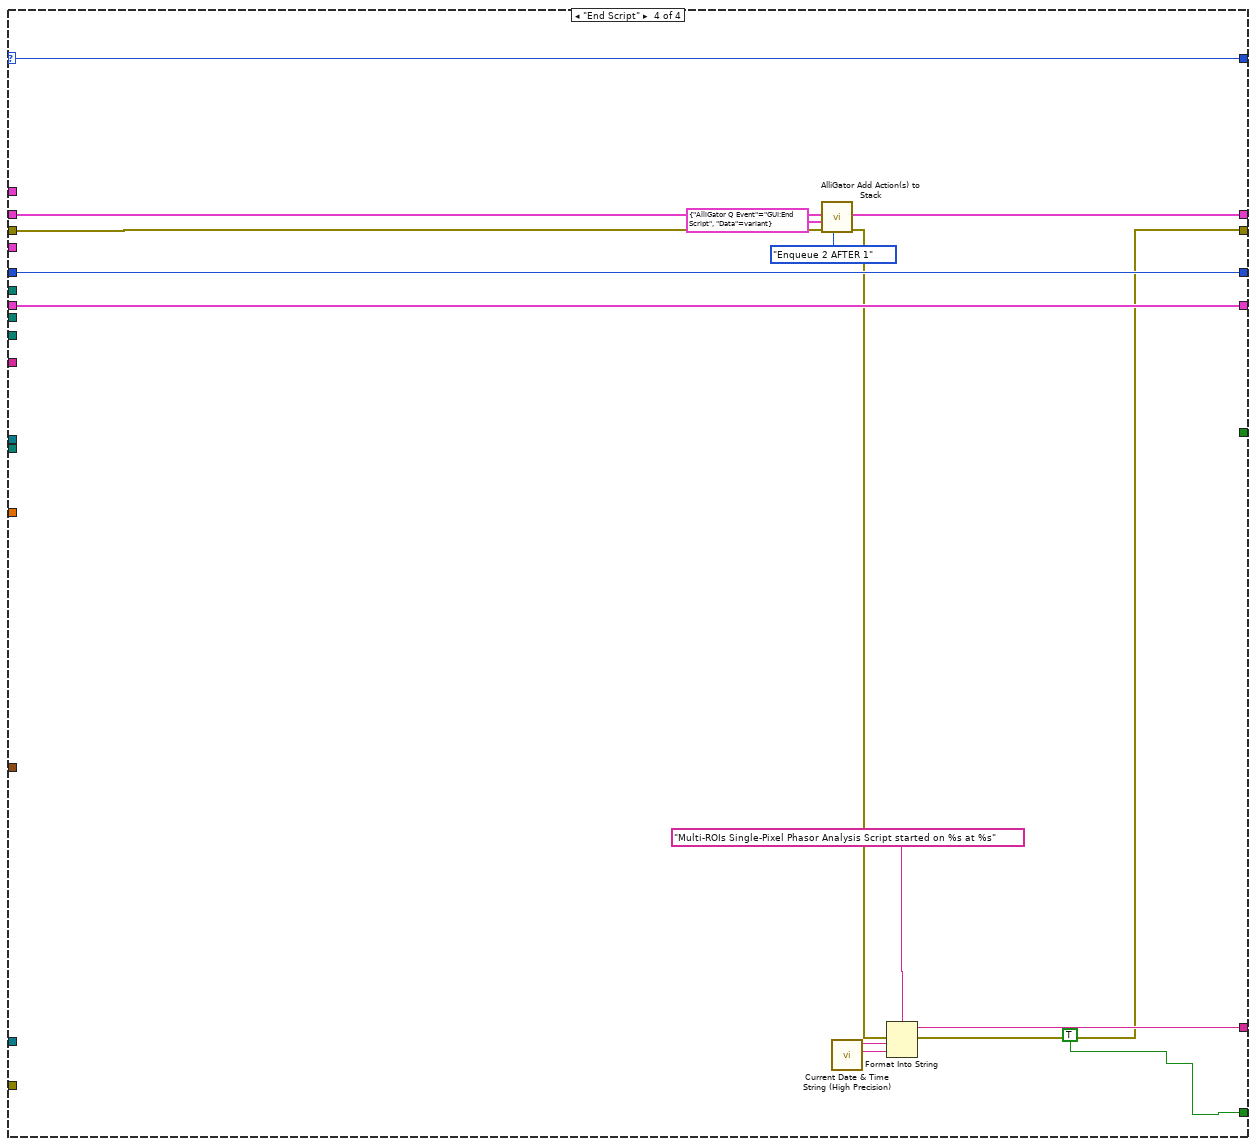
[diagram p15: hidden frame]
diagram:
  w10 = 0  # # ROIs Loaded
  # "Author: Xavier Michalet\nCopyright 2025 REGENTS OF THE UNIVERSITY OF CALIFORNIA\n\nRedistribution and use in source and binary forms, with or without modification, are permitted provided that the following conditions are met:\n\n1. Redistributions of source code must retain the above copyright notice, this list of conditions and the following disclaimer.\n\n2. Redistributions in binary form must reproduce the above copyright notice, this list of conditions and the following disclaimer in the documentation and/or other materials provided with the distribution.\n\n3. Neither the name of the copyright holder nor the names of its contributors may be used to endorse or promote products derived from this software without specific prior written permission.\n\nTHIS SOFTWARE IS PROVIDED BY THE COPYRIGHT HOLDERS AND CONTRIBUTORS “AS IS” AND ANY EXPRESS OR IMPLIED WARRANTIES, INCLUDING, BUT NOT LIMITED TO, THE IMPLIED WARRANTIES OF MERCHANTABILITY AND FITNESS FOR A PARTICULAR PURPOSE ARE DISCLAIMED. IN NO EVENT SHALL THE COPYRIGHT HOLDER OR CONTRIBUTORS BE LIABLE FOR ANY DIRECT, INDIRECT, INCIDENTAL, SPECIAL, EXEMPLARY, OR CONSEQUENTIAL DAMAGES (INCLUDING, BUT NOT LIMITED TO, PROCUREMENT OF SUBSTITUTE GOODS OR SERVICES; LOSS OF USE, DATA, OR PROFITS; OR BUSINESS INTERRUPTION) HOWEVER CAUSED AND ON ANY THEORY OF LIABILITY, WHETHER IN CONTRACT, STRICT LIABILITY, OR TORT (INCLUDING NEGLIGENCE OR OTHERWISE) ARISING IN ANY WAY OUT OF THE USE OF THIS SOFTWARE, EVEN IF ADVISED OF THE POSSIBILITY OF SUCH DAMAGE."
  # "Dataset Loading & Pre-processing Options"
  n1 = call "AlliGator Phasor Frequency.vi"() -> ("Phasor Frequency"=w7:dbl[unit])
  n2 = node(w7) -> (w8:dbl)
  n3 = while {
    shift-right: [w46] -> w13
    shift-left: _ -> [w49]
    shift-right: [w44] -> _
    shift-left: T26."Start Script" -> [w47]
    shift-right: [w42] -> w21
    shift-left: "Alligator Queue Elements in" -> [w48]
    tunnel: "IRF File" -> [w41]
    tunnel: "Phasor Graph refnum" -> [w40]
    tunnel: "ROI File" -> [w39]
    tunnel: "Dataset File" -> [w38]
    tunnel: "Source Image" ("Destination Image") -> [w37]
    shift-right: [w36] -> _
    shift-left: w10 -> [w34]
    tunnel: [w35] -> w12
    tunnel: "Results Folder" -> [w33]
    tunnel: w8 -> [w32]
    tunnel: "Lifetime Graph Refnum" -> [w31]
    tunnel: "Error In" -> [w30]
    shift-right: [w28] -> _
    shift-left: _ -> [w29]
    tunnel: "IRF Loading & Pre-processing Options" -> [w27]
    tunnel: "Dataset Loading & Pre-processing Options" -> [w26]
    tunnel: "Phasor Parameters Scatter Plot" -> [w25]
    tunnel: [w24] -> w1
    stop <- w43 stop-if-true
    n4 = case shown="\"Load & Analyse FLI Dataset: Phasor\"" w47 {
      selector: w47 -> [w58 w80 w216 w327]
      tunnel: w49 -> [_ w75 w207 w324]
      tunnel: w48 -> [w55 w81 w217 w325]
      tunnel: [w52 w78 w214 w314] -> w46
      tunnel: [w58 w80 w216 w327] -> w45
      tunnel: [_ w71 _ TRUE] -> w43
      tunnel: [w53 w79 w215 w323] -> w42
      tunnel: w41 -> [_ w65 _ _]
      tunnel: w40 -> [_ w77 w212 _]
      tunnel: w39 -> [_ w76 w211 _]
      tunnel: w38 -> [_ _ w213 _]
      tunnel: w37 -> [_ w74 _ _]
      tunnel: [w57 w72 w210 w318] -> w36
      tunnel: [_ w70 _ _] -> w35
      tunnel: w34 -> [w57 _ w210 w318]
      tunnel: w33 -> [_ w62 w196 _]
      tunnel: w32 -> [_ _ w209 _]
      tunnel: w31 -> [_ _ w208 _]
      tunnel: w30 -> [w54 _ _ _]
      tunnel: w29 -> [_ w69 w194 w317]
      tunnel: [w56 w68 w194 w317] -> w28
      tunnel: w27 -> [_ w67 _ _]
      tunnel: w26 -> [w56 _ _ _]
      tunnel: w25 -> [_ _ w197 _]
      tunnel: [_ _ _ w316] -> w24
      frame "Start Script", Default {
        n5 = call-poly "AlliGator Add Action(s) to Stack.vi"("Elements Order in Action Stack (Default: 2 BEFORE 1)"=Alligator_Elements_Order_in_Action_Stack."Enqueue 2 AFTER 1", "Error In"=w54, "Alligator Atomic Action"=T23 {"AlliGator Q Event"=enum."GUI:Start Script", "Data"=variant}, "Alligator Queue Element 1"=w55) -> ("Error Out"=w52:errorcluster, "Alligator Queue Element 1 (+ 2)"=w53:T23[])  [unwired: 6 in]
      }
      frame "Load & Analyze IRF Dataset" {
        # "Extract pixel-wise IRFs and phasors, compute calibration map, save related files"
        n6 = call "AlliGator Preview ROI File.vi"("Destination Image"=w74, "File Path"=w76) -> ("Error Out"=w63:errorcluster, "Phasor Plot Image"=w60:bool, "# ROIs Loaded"=w73:i32)  [unwired: 7 in]
        n7 = Unbundle By Name(w63) -> ("status"=w64:bool)
        n8 = Empty String/Path?(string/path=w62) -> (empty?=w61:bool)
        n9 = Empty String/Path?(string/path=w65) -> (empty?=w59:bool)
        n10 = Compound Arithmetic op=AND(invert w60, invert w64) -> (w66:bool)
        n11 = case shown="True" w66 {
          tunnel: w81 -> [w84 w103]
          tunnel: [w84 w102] -> w79
          tunnel: [w82 w101] -> w78
          tunnel: w77 -> [_ w100]
          tunnel: w76 -> [_ w99]
          tunnel: w75 -> [_ w98]
          tunnel: w65 -> [_ w97]
          tunnel: w73 -> [_ w95]
          tunnel: w60 -> [_ w96]
          tunnel: [_ w94] -> w72
          tunnel: [_ w93] -> _
          tunnel: [_ w92] -> w71
          tunnel: [_ w91] -> w70
          tunnel: w62 -> [_ w90]
          tunnel: w69 -> [w83 w89]
          tunnel: [w83 w88] -> w68
          tunnel: w67 -> [_ w87]
          tunnel: w63 -> [w82 _]
          tunnel: w61 -> [_ w86]
          tunnel: w59 -> [_ w85]
          frame False {
            # "Either error in or Phasor Plot Image ROIs"
          }
          frame True {
            n12 = case shown="False" w96 {
              tunnel: w103 -> [w116 w185]
              tunnel: [w115 w185] -> w102
              tunnel: [w114 w179] -> w101
              tunnel: w100 -> [w110 _]
              tunnel: w99 -> [w113 w183]
              tunnel: w98 -> [w108 _]
              tunnel: w97 -> [w112 _]
              tunnel: w95 -> [w111 _]
              tunnel: [w111 _] -> w94
              tunnel: [_ w184] -> w93
              tunnel: [_ TRUE] -> w92
              tunnel: [_ w180] -> w91
              tunnel: w90 -> [w109 _]
              tunnel: w89 -> [w106 w178]
              tunnel: [w106 w178] -> w88
              tunnel: w87 -> [w107 _]
              tunnel: w86 -> [w105 _]
              tunnel: w85 -> [w104 _]
              frame False {
                # "appropriate ROI File: proceed with script"
                n13 = case shown="False" w104 {
                  tunnel: w116 -> [w164 w177]
                  tunnel: [w163 w177] -> w115
                  tunnel: [w162 w176] -> w114
                  tunnel: w113 -> [w161 _]
                  tunnel: w112 -> [w158 _]
                  tunnel: w110 -> [w157 _]
                  tunnel: w109 -> [w156 _]
                  tunnel: w108 -> [w144 w176]
                  tunnel: w107 -> [w140 _]
                  tunnel: w105 -> [w118 _]
                  frame False {
                    w147 = T23 {"AlliGator Q Event"=enum."Phasor Graph:Clear Phasor Graph", "Data"=variant}  # 5. Clear Phasor Graph
                    w124 = T23 {"AlliGator Q Event"=enum."Calibration:Apply Phasor Calibration", "Data"=variant}  # 10. Calibrate IRF Phasors (send them all to (1,0))
                    w125 = T29 {"Multiplot XY Graph"=refnum, "Mouse Coordinates"={"Horizontal"=2147483647, "Vertical"=2147483647}}  # Last Plot
                    w128 = T23 {"AlliGator Q Event"=enum."Calibration:Set Calibration Type", "Data"=variant}  # 9. Set Phasor Calibration to calibration map
                    w133 = T23 {"AlliGator Q Event"=enum."Calibration:Use as Calibration Map", "Data"=variant}  # 7. Use IRF phasors as calibration map
                    w152 = T23 {"AlliGator Q Event"=enum."FLI Dataset:All ROIs Phasor Analysis", "Data"=variant}  # 6. Compute all pixel IRF ROI phasors
                    w135 = T23 {"AlliGator Q Event"=enum."Calibration:Set Calibration Type", "Data"=variant}  # 4. Turn off Phasor Calibration
                    w142 = T23 {"AlliGator Q Event"=enum."Files:Set Dataset Loading & Pre-processing Options", "Data"=variant}  # 1. Set IRF Options
                    w145 = T23 {"AlliGator Q Event"=enum."Files:Load File (all Types)_Scriptable", "Data"=variant}  # 2. Load IRF Dataset
                    # "3. Load ROIs, merge & convert them to single pixel ROIs"
                    # "an IRF File has been provided"
                    n14 = call <vilib>:"Get File Extension.vi"("error in (no error)"=w144, "file"=w158) -> ("error out"=w137:errorcluster, "filename without extension"=w136:string)  [unwired: 5 in, 3 out]
                    n15 = Format Into String(initial string="All ROIs IRFs - " ("format string"), error in=w137, w136) -> (resulting string=w122:string, error out=w120:errorcluster)  [unwired: 1 in]
                    n16 = call <vilib>:"Is Name Multiplatform.vi"("error in (no error)"=w120, "filename"=w122) -> ("error out"=w119:errorcluster, "suggested filename"=w121:string)  [unwired: 5 in, 3 out]
                    n17 = Concatenate Strings(w121, ".calM" ("string")) -> (w131:string)
                    n18 = Build Path(base path=w156, name or relative path=w131) -> (appended path=w130:path)
                    n19 = case "6b. Save  IRF Phasor Plot" shown="False" w118 {
                      tunnel: w157 -> [w175 _]
                      tunnel: w156 -> [w174 _]
                      tunnel: [w173 _] -> w151
                      tunnel: [w172 _] -> w139
                      tunnel: w121 -> [w171 _]
                      tunnel: w119 -> [w170 _]
                      frame False {
                        n20 = call "AlliGator Save Single Phasor Plot Script.vi"("Error In"=w170, "Plot Name"=w171, "Destination Folder path"=w174, "Phasor Graph Refnum"=w175) -> ("Error Out"=w172:errorcluster, "Name & Save Phasor Plot Script"=w173:T23[])  [unwired: 6 in]
                      }
                      frame True {
                      }
                    }
                    n21 = call "Last Plot Mouse Coordinates Constant.vi"() -> ("Selected Plots Mouse Coordinates Equivalent"=w117:T31)
                    n22 = case shown="False" w118 {
                      tunnel: [w169 _] -> w150
                      tunnel: w130 -> [w165 _]
                      frame False {
                        w166 = T34 {"Load/Save"=TRUE, "File Path"=path ""}  # Save
                        w168 = T23 {"AlliGator Q Event"=enum."Calibration:Load/Save Phasor Calibration Map", "Data"=variant}  # 8. Save calibration map
                        n23 = Bundle By Name(cluster=w166, "File Path"=w165) -> (w167:T34)
                        n24 = Bundle By Name(cluster=w168, "Data"=w167) -> (w169:T23)
                      }
                      frame True {
                      }
                    }
                    n25 = Bundle By Name(cluster=w125, "Multiplot XY Graph"=w157, "Mouse Coordinates"=w117) -> (w126:T29)
                    n26 = Bundle By Name(cluster=w142, "Data"=w140) -> (w141:T23)
                    n27 = Bundle By Name(cluster=w145, "Data"=w158) -> (w155:T23)
                    n28 = call "AlliGator Load, Merge & to Pixel ROIs Script.vi"("Error In"=w144, "ROI File"=w161) -> ("Error Out"=w138:errorcluster, "Load & Convert ROIs to pixel ROIs"=w154:T23[])  [unwired: 8 in]
                    n29 = Bundle By Name(cluster=w124, "Data"=-1) -> (w146:T23)
                    n30 = Bundle By Name(cluster=w135, "Data"=Phasor_Calibration_Type."None" ("Calibration Type")) -> (w153:T23)
                    n31 = Bundle By Name(cluster=w128, "Data"=Phasor_Calibration_Type."Phasor Map" ("Calibration Type")) -> (w148:T23)
                    n32 = Bundle By Name(cluster=w133, "Data"=w126) -> (w149:T23)
                    n33 = Merge Errors(w138, w139) -> (w143:errorcluster)
                    n34 = Build Array (concatenate)(w141, w155, w154, w153, w147, w152, w151, w149, w150, w148, w146) -> (w160:T23[])
                    n35 = call-poly "AlliGator Add Action(s) to Stack.vi"("Elements Order in Action Stack (Default: 2 BEFORE 1)"=Alligator_Elements_Order_in_Action_Stack."Enqueue 2 AFTER 1", "Error In"=w143, "Alligator Queue Element 2"=w160, "Alligator Queue Element 1"=w164) -> ("Error Out"=w162:errorcluster, "Alligator Queue Element 1 (+ 2)"=w163:T23[])  [unwired: 6 in]
                  }
                  frame True {
                    # "no IRF file: use current calibration settings"
                  }
                }
              }
              frame True {
                w180 = TRUE  # Error
                # "ROI File is for Phasor Plot"
                n36 = Format Into String(format string="%s is not an Image Source ROI File", w183) -> (resulting string=w184:string)  [unwired: 2 in, 1 out]
                n37 = xnode "Error Ring"() -> ("error out"=w179:errorcluster)
              }
            }
          }
        }
      }
      frame "Load & Analyse FLI Dataset: Phasor" {
        w199 = T23 {"AlliGator Q Event"=enum."Files:Set Dataset Loading & Pre-processing Options", "Data"=variant}  # 1. Set Dataset Options
        w203 = T23 {"AlliGator Q Event"=enum."Files:Load File (all Types)_Scriptable", "Data"=variant}  # 2. Load FLI Dataset
        # "compute calibrated pixel-wise phasors for each ROI,  compute phase lifetimes and save files"
        n38 = Unbundle By Name(w194) -> ("Clear Phasor Graph"=w193:bool)
        n39 = call <vilib>:"Get File Extension.vi"("error in (no error)"=w207, "file"=w213) -> ("error out"=w201:errorcluster, "filename without extension"=w202:string)  [unwired: 5 in, 3 out]
        n40 = Bundle By Name(cluster=w203, "Data"=w213) -> (w204:T23)
        n41 = case shown="True" w193 {
          tunnel: [_ T23 {"AlliGator Q Event"=enum."Phasor Graph:Clear Phasor Graph", "Data"=variant}] -> w191
          frame False {
          }
          frame True {
          }
        }
        n42 = Bundle By Name(cluster=w199, "Data"=w194) -> (w192:T23)
        n43 = call "Last Plot Mouse Coordinates Constant.vi"() -> ("Selected Plots Mouse Coordinates Equivalent"=w190:T31)
        n44 = Empty String/Path?(string/path=w196) -> (empty?=w195:bool)
        n45 = Build Array(w192, w191, w204) -> (w198:T23[])
        n46 = for "3. For Loop on loaded ROIs" {
          N: w210 -> [_]
          shift-right: [w247] -> w206
          shift-left: w198 -> [w248]
          tunnel: w212 -> [w244]
          tunnel: w196 -> [w223]
          tunnel: w202 -> [w228]
          tunnel: w209 -> [w226]
          tunnel: w212 -> [w229]
          tunnel: w211 -> [w241]
          tunnel: w207 -> [w238]
          tunnel: w201 -> [w239]
          tunnel: [w235] -> w200
          tunnel: w208 -> [w222]
          tunnel: w197 -> [w225]
          tunnel: w195 -> [w221]
          tunnel: w190 -> [w219]
          i -> [w242]
          w246 = T23 {"AlliGator Q Event"=enum."FLI Dataset:All ROIs Phasor Analysis", "Data"=variant}  # i2. Compute single pixel phasors
          # "i1. Load all, select one ROI & convert to pixel ROIs"
          # "i3. Save FLI Dataset ROI Phasor Plot"
          n47 = Empty Array?(array=w225) -> (empty?=w220:bool)
          n48 = Increment(x=w242) -> (x+1=w227:i32)
          n49 = Format Into String(format string=" (ROI %d, f = %#g MHz)", initial string=w228, error in=w239, w227, w226) -> (resulting string=w234:string, error out=w233:errorcluster)
          n50 = call <vilib>:"Is Name Multiplatform.vi"("error in (no error)"=w233, "filename"=w234) -> ("error out"=w232:errorcluster, "suggested filename"=w224:string)  [unwired: 5 in, 3 out]
          n51 = case shown="True" w220 {
            tunnel: [w250 w266] -> w230
            tunnel: w229 -> [w251 w265]
            tunnel: w224 -> [_ w264]
            tunnel: w223 -> [_ w263]
            tunnel: w222 -> [_ w262]
            tunnel: w225 -> [_ w261]
            tunnel: w221 -> [_ w260]
            tunnel: w219 -> [w249 w259]
            frame True {
              # "i5. Compute Phase Lifetime Trajectory"
              n52 = disable-structure shown="Disabled" {
                disable-tunnel: w251 -> [w257 _]
                disable-tunnel: [w253 _] -> w250
                disable-tunnel: w249 -> [w252 _]
                frame Disabled {
                  n53 = Bundle By Name(cluster=T29 {"Multiplot XY Graph"=refnum, "Mouse Coordinates"={"Horizontal"=2147483647, "Vertical"=2147483647}} ("Last Plot"), "Mouse Coordinates"=w252, "Multiplot XY Graph"=w257) -> (w254:T29)
                  n54 = Bundle By Name(cluster=T23 {"AlliGator Q Event"=enum."Phasor Graph:Phase Lifetime Trajectory (deprecated)", "Data"=variant}, "Data"=w254) -> (w258:T23)
                  n55 = Build Array(w258) -> (w253:T23[])
                }
                frame Enabled {
                }
              }
            }
            frame False {
              # "i5. Compute Parameter 2 vs Parameter 1 Scatter Plots"
              n56 = for {
                tunnel: [w279] -> w266 mode=concatenating
                tunnel: w265 -> [w275]
                tunnel: w264 -> [w278]
                tunnel: w263 -> [w277]
                tunnel: w262 -> [w276]
                tunnel: w261 -> [w274] mode=indexing
                tunnel: w260 -> [w273]
                tunnel: w259 -> [w267]
                n57 = Unbundle By Name(w274) -> ("Parameter 2"=w272:T2, "Parameter 1"=w271:T2)
                n58 = call "AlliGator Check Valid Scatter Plot Parameters.vi"("Parameter 2"=w271, "Parameter 1"=w272) -> ("Parameter 2"=w269:T2, "Parameter 1"=w270:T2, "Cancelled?"=w268:bool)  [unwired: 6 in, 1 out]
                n59 = case shown="False" w268 {
                  tunnel: [w299 _] -> w279
                  tunnel: w278 -> [w298 _]
                  tunnel: w277 -> [w297 _]
                  tunnel: w276 -> [w296 _]
                  tunnel: w275 -> [w287 _]
                  tunnel: w274 -> [w285 _]
                  tunnel: w273 -> [w284 _]
                  tunnel: w270 -> [w283 _]
                  tunnel: w269 -> [w282 _]
                  tunnel: w267 -> [w280 _]
                  frame False {
                    n60 = Bundle By Name(cluster=T32 {"Multiplot XY Graph"=refnum, "Mouse Coordinates"={"Horizontal"=2147483647, "Vertical"=2147483647}, "Plot Index"=-1} ("Last Plot"), "Mouse Coordinates"=w280, "Multiplot XY Graph"=w287) -> (w288:T32)
                    n61 = Format Into String(format string="_%s vs %s" ("string"), w283, w282) -> (resulting string=w291:string)  [unwired: 2 in, 1 out]
                    n62 = Concatenate Strings(w298, w291) -> (w290:string)
                    n63 = Build Path(base path=w297, name or relative path=w290) -> (appended path=w289:path)
                    n64 = case shown="False" w284 {
                      tunnel: w296 -> [w306 _]
                      tunnel: [w304 _] -> w293
                      tunnel: w289 -> [w301 _]
                      tunnel: w280 -> [w300 _]
                      frame False {
                        n65 = Bundle By Name(cluster=T33 {"XY Graph Refnum"=refnum, "Mouse Coords"={"Horizontal"=2147483647, "Vertical"=2147483647}, "File Path"=path ""} ("Last Plot"), "Mouse Coords"=w300, "XY Graph Refnum"=w306, "File Path"=w301) -> (w303:T33)
                        n66 = Bundle By Name(cluster=T23 {"AlliGator Q Event"=enum."Generic Graph:Save Plot", "Data"=variant} ("element"), "Data"=w303) -> (w304:T23)
                      }
                      frame True {
                      }
                    }
                    n67 = Bundle("Last Plot"=w288, "Scatter Plot"=w285) -> (w286:cluster{"Last Plot":T32, "Scatter Plot":T1})  [unwired: 1 in]
                    n68 = Bundle By Name(cluster=T23 {"AlliGator Q Event"=enum."Phasor Graph:Parameter 2 vs Parameter 1 Scatter Plot", "Data"=variant}, "Data"=w286) -> (w294:T23)
                    n69 = Build Array(w294, w293) -> (w299:T23[])
                  }
                  frame True {
                  }
                }
              }
            }
          }
          n70 = case shown="False" w221 {
            tunnel: [w312 _] -> w245
            tunnel: w244 -> [w311 _]
            tunnel: [w310 w313] -> w236
            tunnel: w232 -> [w309 w313]
            tunnel: w224 -> [w308 _]
            tunnel: w223 -> [w307 _]
            frame False {
              n71 = call "AlliGator Save Single Phasor Plot Script.vi"("Error In"=w309, "Plot Name"=w308, "Destination Folder path"=w307, "Phasor Graph Refnum"=w311) -> ("Error Out"=w310:errorcluster, "Name & Save Phasor Plot Script"=w312:T23[])  [unwired: 6 in]
            }
            frame True {
            }
          }
          n72 = call "AlliGator Load ROIs, Select one ROI (& Convert to Pixel ROIs) Script.vi"("Convert to single Pixel ROIs"=TRUE, "Error In"=w238, "ROI ID"=w227, "ROI File"=w241) -> ("Error Out"=w237:errorcluster, "Load & Convert ID'ed ROI to pixel ROIs"=w240:T23[])  [unwired: 6 in]
          n73 = Merge Errors(w237, w236) -> (w235:errorcluster)
          n74 = Build Array (concatenate)(w248, w240, w246, w245, w230) -> (w247:T23[])
        }
        n75 = call-poly "AlliGator Add Action(s) to Stack.vi"("Elements Order in Action Stack (Default: 2 BEFORE 1)"=Alligator_Elements_Order_in_Action_Stack."Enqueue 2 AFTER 1", "Error In"=w200, "Alligator Queue Element 2"=w206, "Alligator Queue Element 1"=w217) -> ("Error Out"=w214:errorcluster, "Alligator Queue Element 1 (+ 2)"=w215:T23[])  [unwired: 6 in]
      }
      frame "End Script" {
        n76 = call-poly "AlliGator Add Action(s) to Stack.vi"("Elements Order in Action Stack (Default: 2 BEFORE 1)"=Alligator_Elements_Order_in_Action_Stack."Enqueue 2 AFTER 1", "Error In"=w324, "Alligator Atomic Action"=T23 {"AlliGator Q Event"=enum."GUI:End Script", "Data"=variant} ("element"), "Alligator Queue Element 1"=w325) -> ("Error Out"=w315:errorcluster, "Alligator Queue Element 1 (+ 2)"=w323:T23[])  [unwired: 6 in]
        n77 = call "Current Date & Time String (High Precision).vi"() -> ("time string"=w321:string, "date string"=w320:string)  [unwired: 8 in, 2 out]
        n78 = Format Into String(format string="Multi-ROIs Single-Pixel Phasor Analysis Script started on %s at %s" ("initial string"), error in=w315, w320, w321) -> (resulting string=w316:string, error out=w314:errorcluster)  [unwired: 1 in]
      }
    }
    n79 = Increment(x=w45) -> (x+1=w44:T26)
  }
  "Error Out" <- w13
  "Alligator Queue Elements out" <- w21
  "Message" <- w1
  n80 = Not(x=w12) -> (.not. x?=w11:bool)
  n81 = call "Alligator Variables Storage.vi"("Get(F)/Set"=w11, "AlliGator Variable"=AlliGator_Variables_List."GUI:Script in progress" ("Alligator Variable"), "Error In"=w13, "Data in"=TRUE) -> ()  [unwired: 5 in, 3 out]
